vi "keithley_init.vi"(4 "Node (0-64) in":i8 min=0 max=64 step=1, 5 "Limit in":dbl=1.0, 7 "Source Function (Current) 3":enum32{"Current", "Voltage"}(ring)=enum."Voltage", 8 "error in (no error)":errorcluster, 9 "Channel (Channel A) in":T1, 11 "VISA Refnum in":refnum<visa-resource-name>) -> (0 "error out":errorcluster, 1 "Init timer":u32, 2 "Node Out":string, 3 "VISA resource name out":refnum<visa-resource-name>)   [LabVIEW 2012]
uses:
  Keithley 2600 Series/Keithley 2600 Series.lvlib
  Keithley 2600 Series/Public/Channel.ctl
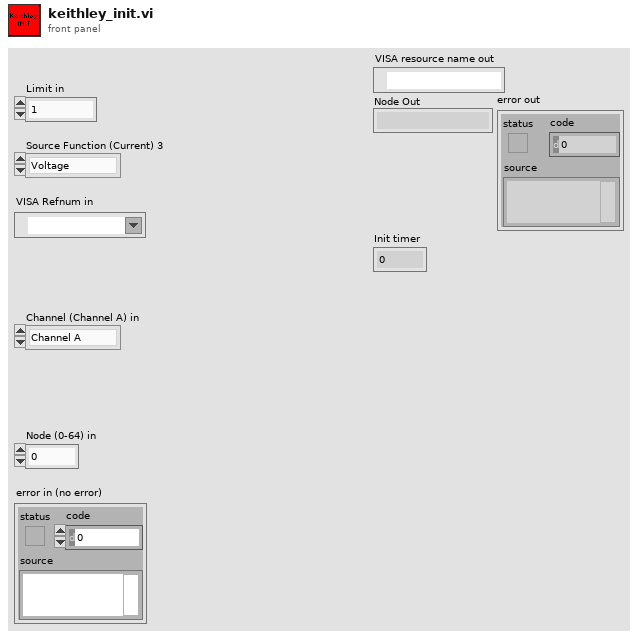
[diagram p1: front panel]
types:
  T1 = typedef "Keithley 2600 Series.lvlib/Channel.ctl" = enum32{"Channel A", "Channel B"}
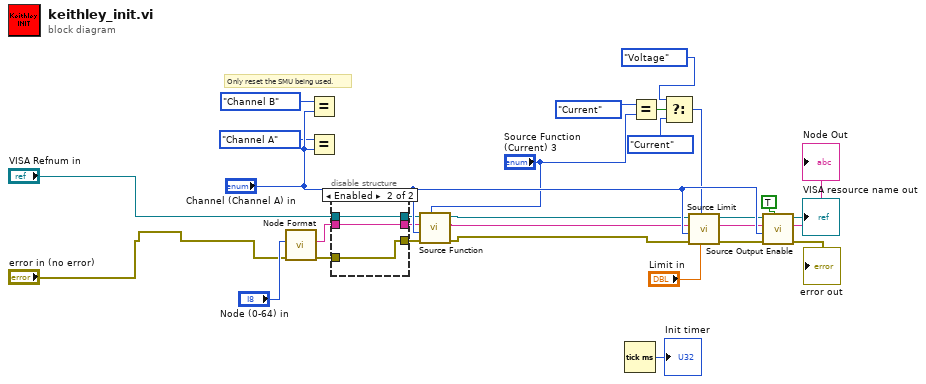
[diagram p0: block diagram]
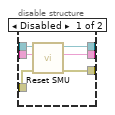
[diagram p2: hidden frame]
diagram:
  # "Only reset the SMU being used."
  n1 = call "Node Format.vi"("error in"="error in (no error)", "Node (0-64)"="Node (0-64) in") -> ("error out"=w10:errorcluster, "Formatted Node"=w11:string)  [unwired: 8 out]
  n2 = Equal?(x=enum32{"Channel A", "Channel B"}."Channel B", y="Channel (Channel A) in") -> ()  [unwired: 1 out]
  n3 = Equal?(x=enum32{"Channel A", "Channel B"}."Channel A", y="Channel (Channel A) in") -> ()  [unwired: 1 out]
  n4 = disable-structure shown="Enabled" {
    disable-tunnel: [w35 w36] -> w14
    disable-tunnel: [w34 w38] -> w13
    disable-tunnel: [w33 w37] -> w12
    disable-tunnel: w11 -> [w32 w37]
    disable-tunnel: w10 -> [w31 w36]
    disable-tunnel: "VISA Refnum in" -> [w30 w38]
    frame Disabled {
      n5 = call "Reset SMU.vi"("error in (no error)"=w31, "Node In"=w32, "VISA resource name"=w30) -> ("error out"=w35:errorcluster, "Node Out"=w33:string, "VISA resource name out"=w34:refnum<visa-resource-name>)  [unwired: 2 in, 4 out]
    }
    frame Enabled {
    }
  }
  n6 = call "Source Function.vi"("Function (Current)"="Source Function (Current) 3", "error in (no error)"=w14, "Channel (Channel A)"="Channel (Channel A) in", "Node In"=w12, "VISA resource name"=w13) -> ("error out"=w28:errorcluster, "Node Out"=w27:string, "VISA resource name out"=w26:refnum<visa-resource-name>)  [unwired: 4 out]
  n7 = Tick Count (ms)() -> (millisecond timer value=→"Init timer":u32)
  n8 = Equal?(x=enum32{"Current", "Voltage"}."Current", y="Source Function (Current) 3") -> (x = y?=w20:bool)
  n9 = Select(t=enum32{"Current", "Voltage"}."Voltage" ("f"), s=w20, f=enum32{"Current", "Voltage"}."Current") -> (s? t:f=w19:enum32{"Current", "Voltage"})
  n10 = call "Source Limit.vi"("Limit (0.000)"="Limit in", "Function (Current)"=w19, "error in (no error)"=w28, "Channel (Channel A)"="Channel (Channel A) in", "Node In"=w27, "VISA resource name"=w26) -> ("error out"=w24:errorcluster, "Node Out"=w22:string, "VISA resource name out"=w25:refnum<visa-resource-name>)  [unwired: 3 out]
  n11 = call "Source Output Enable.vi"("Output (Off)"=TRUE, "error in (no error)"=w24, "Channel (Channel A)"="Channel (Channel A) in", "Node In"=w22, "VISA resource name"=w25) -> ("error out"=→"error out":errorcluster, "Node Out"=→"Node Out":string, "VISA resource name out"=→"VISA resource name out":refnum<visa-resource-name>)  [unwired: 4 out]
